vi "Student t Random.vi"(6 "seed":i32=-1, 7 "reset":bool, 10 "k degrees of freedom":i32=1, 11 "samples":i32=128) -> (0 "error":i32, 3 "Student t random data":dbl[](array[numeric]))   [LabVIEW 2017, in "NI_Gmath.lvlib"]
doc: "Generates random values from a variate X, where X describes the selected distribution type. You must manually select the polymorphic instance to use."
uses:
  <vilib>/gmath/NI_Gmath.lvlib
panel:
  # "Student t Random"
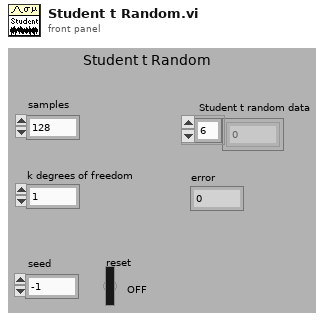
[diagram p1: front panel]
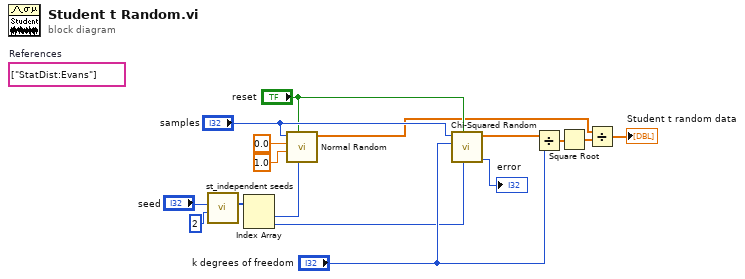
[diagram p0: block diagram]
diagram:
  (unwired) string[] ["StatDist:Evans"]  # References
  n1 = call <vilib>:"st_independent seeds.vi"("number of seeds"=2, "seed"="seed") -> ("independent seeds"=w4:i32[])  [unwired: 9 in]
  n2 = Index Array(array=w4) -> (element #1=w2:i32, element #2=w1:i32)  [unwired: 2 in]
  n3 = call <vilib>:"Normal Random.vi"("seed"=w2, "reset"="reset", "std"=1.0 ("xmax"), "mean"=0.0 ("xmin"), "samples"="samples") -> ("normal random data"=w10:dbl[])  [unwired: 5 in, 1 out]
  n4 = call <vilib>:"Chi-Squared Random.vi"("seed"=w1, "reset"="reset", "k"="k degrees of freedom", "samples"="samples") -> ("error"=→"error":i32, "chi-squared random data"=w12:dbl[])  [unwired: 6 in]
  n5 = Divide(x=w12, y="k degrees of freedom") -> (x/y=w7:dbl[])
  n6 = Square Root(x=w7) -> (sqrt(x)=w6:dbl[])
  n7 = Divide(x=w10, y=w6) -> (x/y=→"Student t random data":dbl[])
